vi "Sweep VWL SET.vi"(6 "Other Fixed Voltage (V)":dbl, 10 "Pulse Width (us)":dbl, 11 "Sweep outfile":path) -> (1 "final current (A)":dbl, 2 "final resistance (ohm)":dbl, 3 "final voltage (V)":dbl)   [LabVIEW 2019]
uses:
  Globals.vi
  <vilib>/Utility/file.llb/Write Delimited Spreadsheet (DBL).vi
panel:
  out "initial resistance (ohm)":dbl format="%#_6p"
  out "VSL (V)":dbl
  out "VBL (V)":dbl
  out "error out":errorcluster
  in  "error in (no error)":errorcluster
  out "VWL (V)":dbl
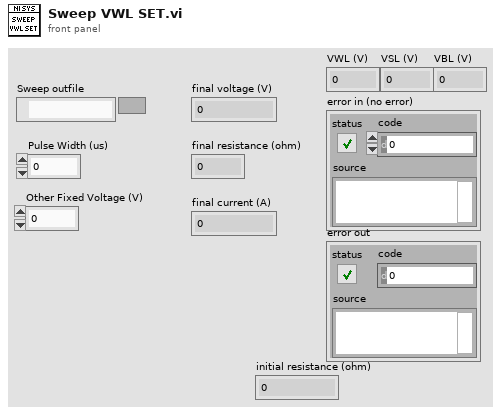
[diagram p1: front panel]
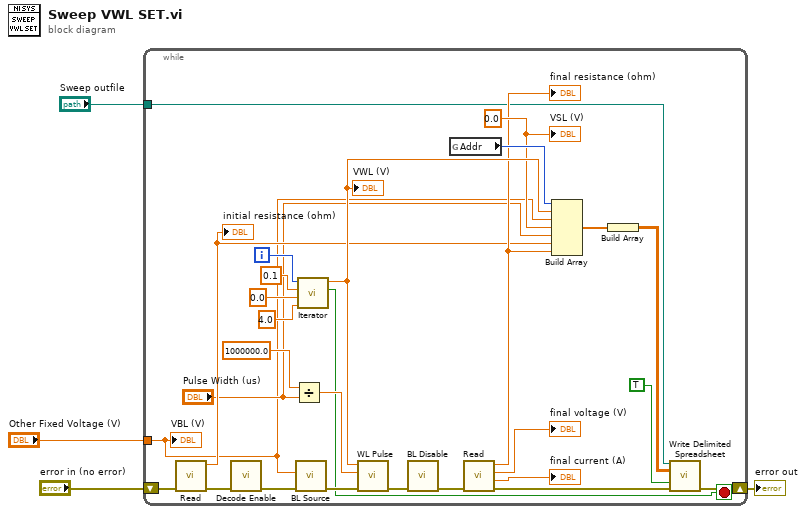
[diagram p0: block diagram]
diagram:
  n1 = while {
    tunnel: "Other Fixed Voltage (V)" -> [w11]
    shift-right: [w6] -> w1
    shift-left: "error in (no error)" -> [w22]
    tunnel: "Sweep outfile" -> [w10]
    i -> [w29]
    stop <- w14 stop-if-true
    w18 = 0.0 ("VSL (V)")
    n2 = call "Read.vi"("error in (no error)"=w22) -> ("error out"=w21:errorcluster, "resistance (ohm)"=w13:dbl)  [unwired: 7 in, 2 out]
    "initial resistance (ohm)" <- w13
    n3 = call "Decode Enable.vi"("error in (no error)"=w21) -> ("error out"=w28:errorcluster)  [unwired: 10 in]
    n4 = Divide(x=1000000.0 ("Sample Rate"), y="Pulse Width (us)") -> (x/y=w24:dbl)
    n5 = call "BL Source.vi"("error in (no error)"=w28, "voltage level (V)"=w11) -> ("error out"=w26:errorcluster)  [unwired: 9 in]
    n6 = call "Iterator.vi"("Final Value"=4.0, "Initial Value"=0.0, "Step"=0.1, "i"=w29) -> ("End Loop"=w14:bool, "Current Value"=w19:dbl)  [unwired: 6 in]
    "VWL (V)" <- w19
    n7 = call "WL Pulse.vi"("error in (no error)"=w26, "Sample Rate"=w24, "VWL (V)"=w19) -> ("error out"=w27:errorcluster)  [unwired: 8 in]
    n8 = call "BL Disable.vi"("error in (no error)"=w27) -> ("error out"=w25:errorcluster)  [unwired: 10 in]
    n9 = global read "Globals.vi" "Addr"() -> (w20:u16)
    n10 = call "Read.vi"("error in (no error)"=w25) -> ("error out"=w9:errorcluster, "current (A)"=→"final current (A)":dbl, "read voltage (V)"=→"final voltage (V)":dbl, "resistance (ohm)"=w15:dbl)  [unwired: 7 in]
    "final resistance (ohm)" <- w15
    n11 = Build Array(w20, w19, w11, w18, "Pulse Width (us)", w13, w15) -> (w8:dbl[])
    n12 = Build Array(w8) -> (w7:dbl[][])
    n13 = call-poly <vilib>:"Write Delimited Spreadsheet.vi"("file path (dialog if empty)"=w10, "2D data"=w7, "append to file? (new file:F)"=TRUE, "error in (no error)"=w9) -> ("error out"=w6:errorcluster)  [unwired: 10 in, 1 out]
    "VSL (V)" <- w18
    "VBL (V)" <- w11
  }
  "error out" <- w1
